vi "Configure Scaling.vi"(0 "VISA resource name":refnum<visa-resource-name>, 1 "Scaling (T: Enable)":bool=TRUE, 2 "Element (0: All)":i32(ring) items=["All", "1", "2", "3", "4", "5", "6"], 5 "VT Ratio (1.0000)":dbl=1.0 min=0.0001 max=99999.9999 format="%.4g", 7 "CT Ratio (1.0000)":dbl=1.0 min=0.0001 max=99999.9999 format="%.4g", 9 "Power Coefficient (1.0000)":dbl=1.0 min=0.0001 max=99999.9999 format="%.4g", 11 "error in (no error)":errorcluster) -> (4 "VISA resource name out":refnum<visa-resource-name>, 15 "error out":errorcluster)   [LabVIEW 2021, in "Yokogawa WT1800 Series.lvlib"]
doc: "Configures the scaling features."
uses:
  <instrlib>/Yokogawa WT1800 Series/Yokogawa WT1800 Series.lvlib
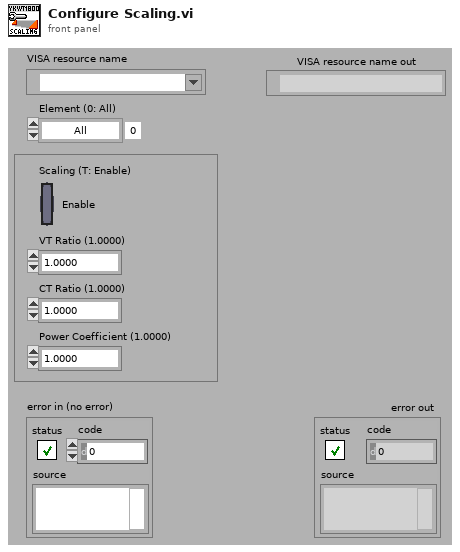
[diagram p1: front panel]
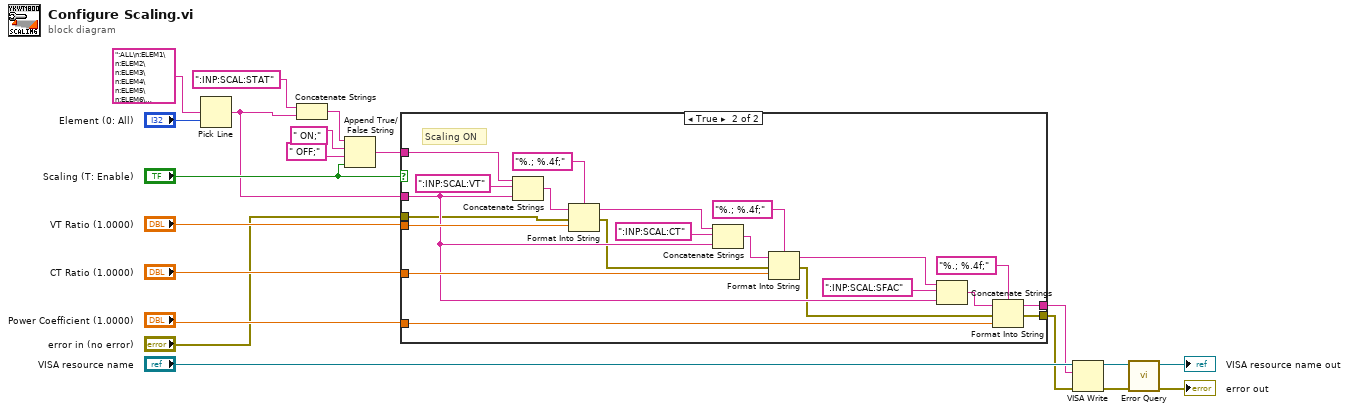
[diagram p0: block diagram]
diagram:
  n1 = Pick Line ("ライン選択")(multi-line string=":ALL\n:ELEM1\n:ELEM2\n:ELEM3\n:ELEM4\n:ELEM5\n:ELEM6\n:SIGMA\n:SIGMB\n:SIGMC" ("複数行文字列"), line index="Element (0: All)") -> (output string=w7:string)  [unwired: 1 in]
  n2 = Concatenate Strings(":INP:SCAL:STAT", w7) -> (w15:string)
  n3 = Append True/False String ("True/False 文字列を追加")(1:"Scaling (T: Enable)", 2:" OFF;", 3:" ON;", 4:w15) -> (0:w9:string)
  n4 = case "ケースストラクチャ" shown="True" "Scaling (T: Enable)" {
    tunnel: w9 -> [w22 w41]
    tunnel: w7 -> [_ w29]
    tunnel: "VT Ratio (1.0000)" -> [_ w39]
    tunnel: "CT Ratio (1.0000)" -> [_ w34]
    tunnel: "Power Coefficient (1.0000)" -> [_ w28]
    tunnel: "error in (no error)" -> [w21 w25]
    tunnel: [w22 w24] -> w2
    tunnel: [w21 w23] -> w1
    frame False {
      # "Scaling OFF"
    }
    frame True {
      # "Scaling ON"
      n5 = Concatenate Strings(w41, ":INP:SCAL:VT", w29) -> (w40:string)
      n6 = Format Into String ("文字列にフォーマット")(format string="%.; %.4f;" ("形式文字列"), initial string=w40, error in=w25, w39) -> (resulting string=w35:string, error out=w26:errorcluster)
      n7 = Concatenate Strings(w35, ":INP:SCAL:CT", w29) -> (w38:string)
      n8 = Format Into String ("文字列にフォーマット")(format string="%.; %.4f;" ("形式文字列"), initial string=w38, error in=w26, w34) -> (resulting string=w30:string, error out=w27:errorcluster)
      n9 = Concatenate Strings(w30, ":INP:SCAL:SFAC", w29) -> (w31:string)
      n10 = Format Into String ("文字列にフォーマット")(format string="%.; %.4f;" ("形式文字列"), initial string=w31, error in=w27, w28) -> (resulting string=w24:string, error out=w23:errorcluster)
    }
  }
  n11 = VISA Write ("VISA書き込み")(VISA resource name="VISA resource name", write buffer=w2, error in (no error)=w1) -> (VISA resource name out=w20:refnum<visa-resource-name>, error out=w19:errorcluster)  [unwired: 1 out]
  n12 = call <instrlib>:"Error Query.vi"("error in (no error)"=w19, "VISA resource name"=w20) -> ("error out"=→"error out":errorcluster, "VISA resource name out"=→"VISA resource name out":refnum<visa-resource-name>)  [unwired: 6 in, 2 out]
